vi "Write Force Measured.vi"(10 "Force Measured":T1 min=-888.0 max=888.0 format="%.2f", 11 "StiffnessMonitor in":refnum<class "StiffnessMonitor.lvclass">) -> (3 "StiffnessMonitor out":refnum<class "StiffnessMonitor.lvclass">)   [LabVIEW 2013, in "StiffnessMonitor.lvclass"]
uses:
  StiffnessMonitor.lvclass
  Typedefs/ForceDemand.ctl
  StiffnessMonitor.lvclass/StiffnessMonitor.ctl
  Typedefs/M2AADTTypedefs.lvlib
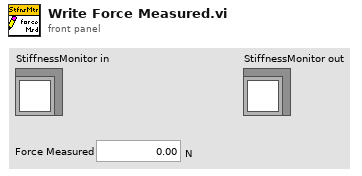
[diagram p1: front panel]
types:
  T1 = typedef "M2AADTTypedefs.lvlib/ForceDemand.ctl" = dbl[unit]
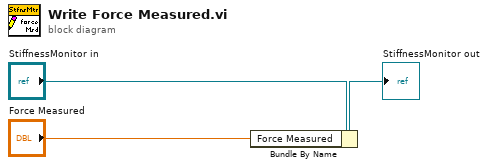
[diagram p0: block diagram]
diagram:
  n1 = Bundle By Name(cluster="StiffnessMonitor in", "Force Measured"="Force Measured") -> (→"StiffnessMonitor out":refnum<class "StiffnessMonitor.lvclass">)
